vi "Child Node Copy.vi"(8 "error in (no error)":errorcluster, 9 "Child In":refnum<class "System Actor.lvclass">, 11 "Ancestor In":refnum<class "Node Actor.lvclass">) -> (0 "error out":errorcluster, 3 "Child Out":refnum<class "System Actor.lvclass">)   [LabVIEW 2024, in "Node Actor.lvclass"]
uses:
  Node Actor.lvclass
  Node Actor.lvclass/Node Actor.ctl
  Root Actor/Root Actor.lvclass
  System Actor/System Actor.lvclass
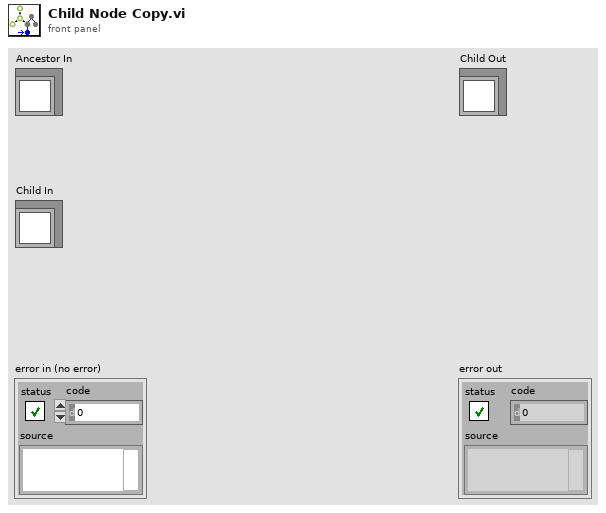
[diagram p1: front panel]
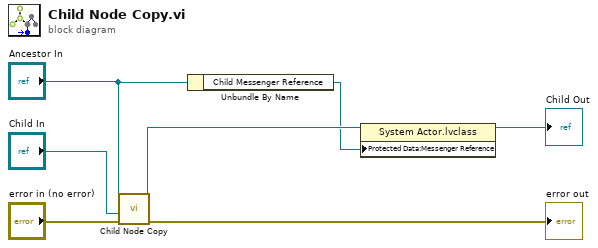
[diagram p0: block diagram]
diagram:
  n1 = call-parent "Child Node Copy.vi"("error in (no error)"="error in (no error)", "Child In"="Child In", "Ancestor In"="Ancestor In") -> ("error out"=→"error out":errorcluster, "Child Out"=w3:refnum<class "System Actor.lvclass">)  [unwired: 7 in]
  n2 = Unbundle By Name("Ancestor In") -> ("Child Messenger Reference"=w1:refnum<data-value>)
  n3 = property class="System Actor.lvclass"(reference=w3, "Protected Data:Messenger Reference"=w1) -> (reference out=→"Child Out":refnum<class "System Actor.lvclass">)  [unwired: 1 in, 1 out]
